vi "Read Buffer.vi"(6 "wait for reply (T)":bool=TRUE, 8 "error in":errorcluster, 10 "pre-read delay":i16=-1, 11 "Module ID":i32=-1) -> (0 "error out":errorcluster, 1 "timed out?":bool, 2 "bytes count":i16, 3 "buffer output":string)   [LabVIEW 2022 SP3, in "Serial-Com-Module.lvlib"]
doc: "It will read the data in the serial port buffer\n_____\nCreated using DQMH Event Scripter 6.1.0.128."
uses:
  Serial-Com-Module.lvlib
  Read Buffer Argument--cluster.ctl
  Read Buffer (Reply Payload)--cluster.ctl
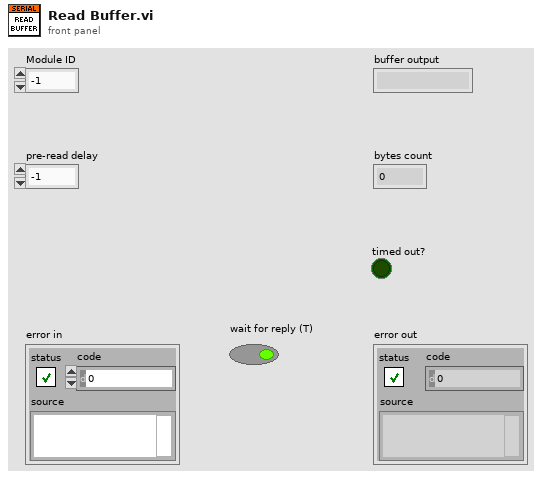
[diagram p1: front panel]
types:
  T1 = typedef "Serial-Com-Module.lvlib/Read Buffer Argument--cluster.ctl" = cluster{"Module ID":i32, "pre-read delay":i16, "Wait Notifier":refnum<notifier>, "wait for reply":bool}
  T2 = typedef "Serial-Com-Module.lvlib/Request Events--cluster.ctl" = cluster{"Stop Module":refnum<user-event>, "Show Panel":refnum<user-event>, "Hide Panel":refnum<user-event>, "Show Diagram":refnum<user-event>, "Get Module Execution Status":refnum<user-event>, "Init Serial":refnum<user-event>, "Open Port":refnum<user-event>, "Close Port":refnum<user-event>, "Read Buffer":refnum<user-event>, "Send":refnum<user-event>, "Send Line":refnum<user-event>, "Send and Receive":refnum<user-event>}
  T3 = typedef "Serial-Com-Module.lvlib/Read Buffer (Reply Payload)--cluster.ctl" = cluster{"buffer output":string, "bytes count":i16, "error":errorcluster}
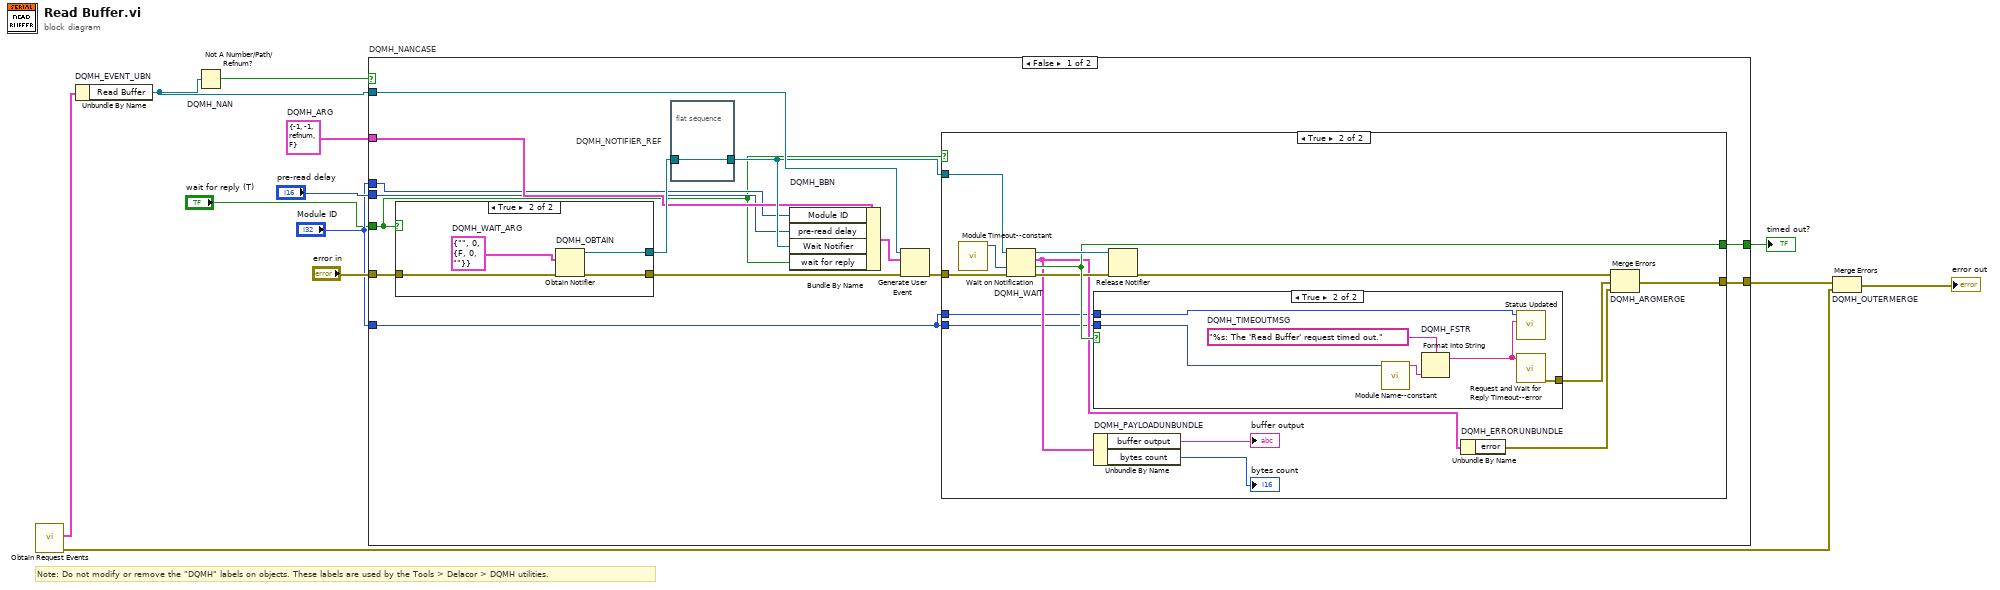
[diagram p0: block diagram]
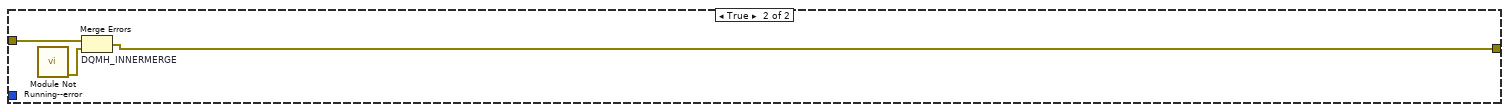
[diagram p5: hidden frame]
diagram:
  w6 = T1 {"Module ID"=-1, "pre-read delay"=-1, "Wait Notifier"=refnum, "wait for reply"=FALSE}  # DQMH_ARG
  # "Note: Do not modify or remove the \"DQMH\" labels on objects. These labels are used by the Tools > Delacor > DQMH utilities."
  n1 = call "Obtain Request Events.vi"() -> ("error out"=w2:errorcluster, "Serial-Com-Module Request Events"=w1:T2)  [unwired: 10 in]
  n2 = Unbundle By Name "DQMH_EVENT_UBN"(w1) -> ("Read Buffer"=w10:refnum<user-event>)
  n3 = Not A Number/Path/Refnum? "DQMH_NAN"(number/path/refnum=w10) -> (NaN/Path/Refnum?=w9:bool)
  n4 = case "DQMH_NANCASE" shown="False" w9 {
    tunnel: "error in" -> [w26 w57]
    tunnel: w10 -> [w24 _]
    tunnel: [w21 w56] -> w7
    tunnel: [w22 _] -> w8
    tunnel: w6 -> [w17 _]
    tunnel: "Module ID" -> [w16 _]
    tunnel: "pre-read delay" -> [w15 _]
    tunnel: "Module ID" -> [w14 _]
    tunnel: "wait for reply (T)" -> [w13 _]
    frame False {
      n5 = case shown="True" w13 {
        tunnel: w26 -> [w50 w54]
        tunnel: [w50 w53] -> w23
        tunnel: [_ w51] -> w19
        frame False {
        }
        frame True {
          w52 = T3 {"buffer output"="", "bytes count"=0, "error"={"status"=FALSE, "code"=0, "source"=""}}  # DQMH_WAIT_ARG
          n6 = Obtain Notifier "DQMH_OBTAIN"(notification data type=w52, error in (no error)=w54) -> (notifier out=w51:refnum<notifier>, error out=w53:errorcluster)  [unwired: 2 in, 1 out]
        }
      }
      n7 = flat-sequence "DQMH_NOTIFIER_REF" {
        tunnel: w19 -> [w27]
        tunnel: [w27] -> w18
        frame #0 {
        }
      }
      n8 = Bundle By Name "DQMH_BBN"(cluster=w17, "Module ID"=w16, "pre-read delay"=w15, "Wait Notifier"=w18, "wait for reply"=w13) -> (w20:T1)
      n9 = Generate User Event(user event=w24, event data cluster=w20, error in=w23) -> (error out=w25:errorcluster)  [unwired: 1 in, 1 out]
      n10 = case shown="True" w13 {
        tunnel: w25 -> [w28 w43]
        tunnel: w18 -> [_ w42]
        tunnel: [_ w40] -> w22
        tunnel: [w28 w39] -> w21
        tunnel: w14 -> [_ w30]
        tunnel: w14 -> [_ w29]
        frame False {
        }
        frame True {
          n11 = call "Module Timeout--constant.vi"() -> ("Module Timeout"=w33:i32)  [unwired: 11 in]
          n12 = Wait on Notification "DQMH_WAIT"(notifier=w42, timeout in ms (-1)=w33, error in (no error)=w43) -> (notifier out=w41:refnum<notifier>, notification=w34:T3, timed out?=w40:bool, error out=w38:errorcluster)  [unwired: 1 in]
          n13 = case shown="True" w40 {
            tunnel: [_ w47] -> w35
            tunnel: w30 -> [_ w45]
            tunnel: w29 -> [_ w44]
            frame False {
            }
            frame True {
              w49 = "%s: The 'Read Buffer' request timed out."  # DQMH_TIMEOUTMSG
              n14 = call "Module Name--constant.vi"("Module ID"=w44) -> ("Module Name"=w46:string)  [unwired: 10 in]
              n15 = Format Into String "DQMH_FSTR"(format string=w49, w46) -> (resulting string=w48:string)  [unwired: 2 in, 1 out]
              n16 = call "Status Updated.vi"("Status"=w48, "Module ID"=w45) -> ()  [unwired: 9 in, 1 out]
              n17 = call "Request and Wait for Reply Timeout--error.vi"("Error Message"=w48) -> ("error out"=w47:errorcluster)  [unwired: 10 in]
            }
          }
          n18 = Unbundle By Name "DQMH_PAYLOADUNBUNDLE"(w34) -> ("buffer output"=→"buffer output":string, "bytes count"=→"bytes count":i16)
          n19 = Release Notifier(notifier=w41, error in (no error)=w38) -> (error out=w37:errorcluster)  [unwired: 1 in, 2 out]
          n20 = Unbundle By Name "DQMH_ERRORUNBUNDLE"(w34) -> ("error"=w36:errorcluster)
          n21 = Merge Errors "DQMH_ARGMERGE"(w37, w35, w36) -> (w39:errorcluster)
        }
      }
    }
    frame True {
      n22 = call "Module Not Running--error.vi"() -> ("error out"=w55:errorcluster)  [unwired: 11 in]
      n23 = Merge Errors "DQMH_INNERMERGE"(w57, w55) -> (w56:errorcluster)
    }
  }
  "timed out?" <- w8
  n24 = Merge Errors "DQMH_OUTERMERGE"(w7, w2) -> (→"error out":errorcluster)
